vi "buildWorkerConfigure.vi"(8 "error in (no error)":errorcluster, 11 "BuildServer in":refnum<class "BuildServer.lvclass">) -> (0 "error out":errorcluster, 3 "BuildServer out":refnum<class "BuildServer.lvclass">)   [LabVIEW 2017, in "BuildServer.lvlib" / "BuildServer.lvclass"]
uses:
  BuildServer.lvclass
  Volumes/Data/Users/benji667/Git/BuildFarm/src/LabVIEW/vi.lib/BenjaminR/Build Farm/Actors/Framework/Actor wUI/Actor wUI.lvclass
  Classes/BuildWorker Interface/BuildWorker/BuildWorker.lvclass
  BuildServer.lvclass/BuildServer.ctl
  Framework/Actor wUI/Get Config File Name.vi
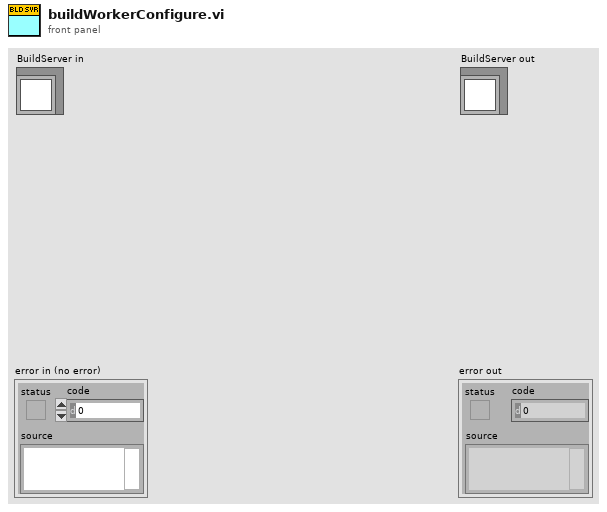
[diagram p1: front panel]
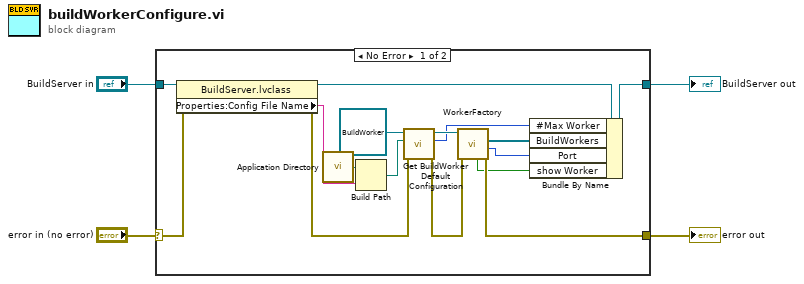
[diagram p0: block diagram]
diagram:
  n1 = case shown="No Error" "error in (no error)" {
    selector: "error in (no error)" -> [w6 w22]
    tunnel: [w13 w22] -> w3
    tunnel: [w19 w21] -> w1
    tunnel: "BuildServer in" -> [w20 w21]
    frame No Error {
      n2 = property class="BuildServer.lvclass"(reference=w20, error in=w6) -> (reference out=w8:refnum<class "BuildServer.lvclass">, error out=w5:errorcluster, "Properties:Config File Name"=w7:string)
      n3 = call <vilib>:"Application Directory.vi"() -> ("Application Directory"=w10:path)
      n4 = Build Path(base path=w10, name or relative path=w7) -> (appended path=w9:path)
      n5 = call-dynamic "Get BuildWorker Default Configuration.vi"("error in (no error)"=w5, "configuration file path"=w9, "BuildWorker in"=refnum<class "BuildWorker.lvclass"> refnum ("BuildWorker Controller in")) -> ("error out"=w14:errorcluster, "#Max Worker"=w16:i32, "BuildWorker out"=w17:refnum<class "BuildWorker.lvclass">)  [unwired: 6 in]
      n6 = call "WorkerFactory.vi"("error in (no error)"=w14, "BuildWorker in"=w17) -> ("error out"=w13:errorcluster, "Port"=w12:u16, "BuildWorkers"=w15:refnum<class "BuildWorker.lvclass">[], "Show"=w11:bool)  [unwired: 5 in, 1 out]
      n7 = Bundle By Name(cluster=w8, "#Max Worker"=w16, "BuildWorkers"=w15, "Port"=w12, "show Worker"=w11) -> (w19:refnum<class "BuildServer.lvclass">)
    }
    frame Error {
    }
  }
  "error out" <- w3
  "BuildServer out" <- w1
